vi "regexINISectionContent.vi"(8 "error in (no error)":errorcluster, 9 "Section Content":string, 10 "Section Name":string) -> (0 "error out":errorcluster, 1 "KVPs":cluster{"key":string, "value":string}[](array[cluster]), 2 "Section Name dup":string, 4 "Comments":string[](array[string]))   [LabVIEW 2013, in "CfgManager.Text.lvlib" / "ConfigManager.Text.INI.lvclass"]
uses:
  ConfigManager.Text.INI.lvclass
  <vilib>/regexp/Match Regular Expression.xnode
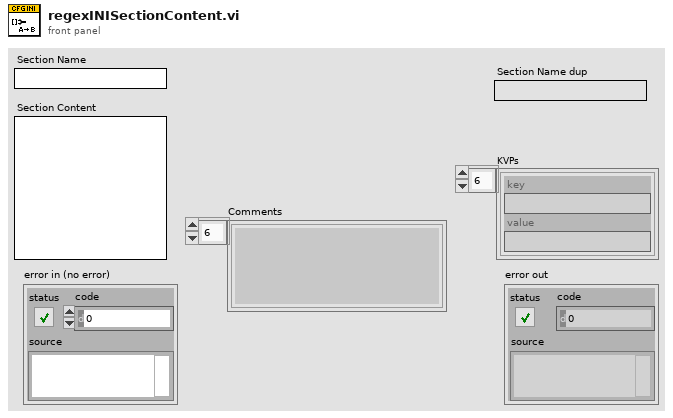
[diagram p1: front panel]
types:
  T1 = cluster{"trimmed string":string, "before match":string}
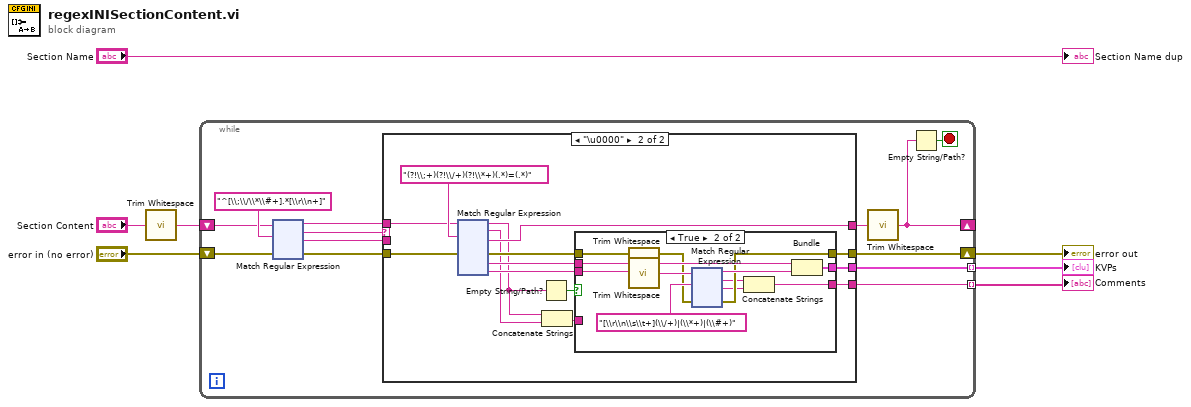
[diagram p0: block diagram]
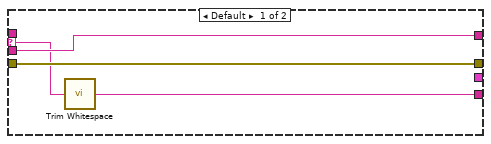
[diagram p2: hidden frame]
diagram:
  n1 = call <vilib>:"Trim Whitespace.vi"("string"="Section Content") -> ("trimmed string"=w2:string)  [unwired: 1 in]
  n2 = while {
    shift-right: [w17] -> _
    shift-left: w2 -> [w8]
    tunnel: [w20] -> w4 mode=indexing
    shift-right: [w16] -> w5
    shift-left: "error in (no error)" -> [w13]
    tunnel: [w15] -> w1 mode=indexing
    stop <- w19 stop-if-true
    n3 = xnode "Match Regular Expression"("input string"=w8, "regular expression"="^[\\;\\/\\*\\#+].*[\\r\\n+]" ("input string"), "error in"=w13) -> ("before match"=w9:string, "whole match"=w10:string, "after match"=w11:string, "error out"=w12:errorcluster)  [unwired: 3 in, 1 out]
    n4 = case shown="\"\"" w10 {
      selector: w10 -> [w22 _]
      tunnel: [_ w35] -> w20
      tunnel: [w24 w34] -> w18
      tunnel: [w23 w32] -> w16
      tunnel: [w21 w30] -> w15
      tunnel: w11 -> [w24 _]
      tunnel: w12 -> [w23 w26]
      tunnel: w9 -> [_ w25]
      frame Default {
        n5 = call <vilib>:"Trim Whitespace.vi"("string"=w22) -> ("trimmed string"=w21:string)  [unwired: 1 in]
      }
      frame "\u0000" {
        n6 = xnode "Match Regular Expression"("input string"=w25, "regular expression"="(?!\\;+)(?!\\/+)(?!\\*+)(.*)=(.*)" ("input string"), "error in"=w26) -> ("before match"=w29:string, "whole match"=w28:string, "after match"=w34:string, "error out"=w33:errorcluster, "submatch 1"=w37:string, "submatch 2"=w36:string)  [unwired: 3 in, 1 out]
        n7 = Empty String/Path?(string/path=w29) -> (empty?=w31:bool)
        n8 = Concatenate Strings(w29, w28) -> (w27:string)
        n9 = case shown="True" w31 {
          tunnel: w37 -> [_ w52]
          tunnel: w36 -> [_ w51]
          tunnel: [_ w50] -> w35
          tunnel: w33 -> [w40 w45]
          tunnel: [w40 w44] -> w32
          tunnel: [w39 w41] -> w30
          tunnel: w27 -> [w39 _]
          frame False {
          }
          frame True {
            n10 = call <vilib>:"Trim Whitespace.vi"("string"=w52) -> ("trimmed string"=w49:string)  [unwired: 1 in]
            n11 = call <vilib>:"Trim Whitespace.vi"("string"=w51) -> ("trimmed string"=w48:string)  [unwired: 1 in]
            n12 = xnode "Match Regular Expression"("input string"=w48, "regular expression"="[\\r\\n\\s\\t+](\\/+)|(\\*+)|(\\#+)" ("input string"), "error in"=w45) -> ("before match"=w47:string, "whole match"=w43:string, "after match"=w42:string, "error out"=w44:errorcluster)  [unwired: 3 in, 1 out]
            n13 = Concatenate Strings(w43, w42) -> (w41:string)
            n14 = Bundle("trimmed string"=w49, "before match"=w47) -> (w50:T1)  [unwired: 1 in]
          }
        }
      }
    }
    n15 = call <vilib>:"Trim Whitespace.vi"("string"=w18) -> ("trimmed string"=w17:string)  [unwired: 1 in]
    n16 = Empty String/Path?(string/path=w17) -> (empty?=w19:bool)
  }
  "KVPs" <- w4
  "error out" <- w5
  "Comments" <- w1
  "Section Name dup" <- "Section Name"
